vi "Constants.vi"   [LabVIEW 2017, in "DSF Core.lvlib" / "DSF PXImc Transceiver.lvclass"]
uses:
  DSF PXImc Transceiver.lvclass
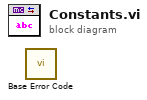
[diagram p0: block diagram]
diagram:
  n1 = call "Base Error Code.vi"() -> ()  [unwired: 11 in, 1 out]
